vi "Base ByRef Ex.vi"() -> ()   [LabVIEW 2020]
uses:
  ByRef Base/ByRef Base.lvclass
panel:
  out "Slide 2":dbl(slide) scale=0.0..10.0
  in  "Slide":dbl(slide) scale=0.0..10.0
  in  "Stop":bool
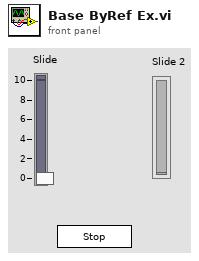
[diagram p1: front panel]
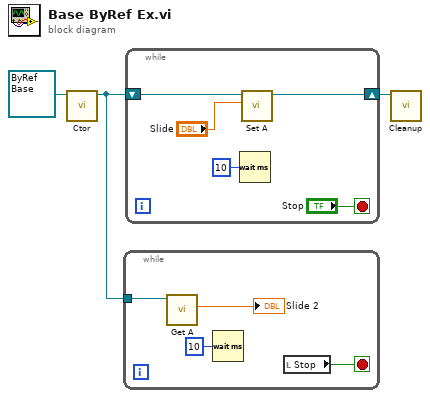
[diagram p0: block diagram]
diagram:
  n1 = call-dynamic "Ctor.vi"("ByRef Base in"=refnum<class "ByRef Base.lvclass"> refnum ("ByRef Base.lvclass")) -> ("ByRef Base out"=w3:refnum<class "ByRef Base.lvclass">)  [unwired: 9 in, 1 out]
  n2 = while {
    tunnel: w3 -> [w7]
    stop <- w5 stop-if-true
    n3 = call "Get A.vi"("ByRef Base in"=w7) -> ("Numeric"=→"Slide 2":dbl)  [unwired: 8 in, 2 out]
    n4 = Wait (ms)(milliseconds to wait=u32 10) -> ()  [unwired: 1 out]
    n5 = local read "Stop"() -> (w5:bool)
  }
  n6 = while {
    shift-right: [w10] -> w2
    shift-left: w3 -> [w11]
    stop <- "Stop" stop-if-true
    n7 = Wait (ms)(milliseconds to wait=u32 10) -> ()  [unwired: 1 out]
    n8 = call "Set A.vi"("Numeric"="Slide", "ByRef Base in"=w11) -> ("ByRef Base out"=w10:refnum<class "ByRef Base.lvclass">)  [unwired: 8 in, 1 out]
  }
  n9 = call-dynamic "Cleanup.vi"("ByRef Base in"=w2) -> ()  [unwired: 10 in, 1 out]
